vi "OpenMV.vi"(7 "JPG":refnum<vi>, 10 "queueName":string="PV_script", 11 "Console Reference":refnum<vi>) -> ()   [LabVIEW 2022 SP3]
panel:
  in  "Grab":bool
  in  "Snap":bool
  out "Image":picture
  out "Plots":T1
  in  "start":bool
  # "Camera View"
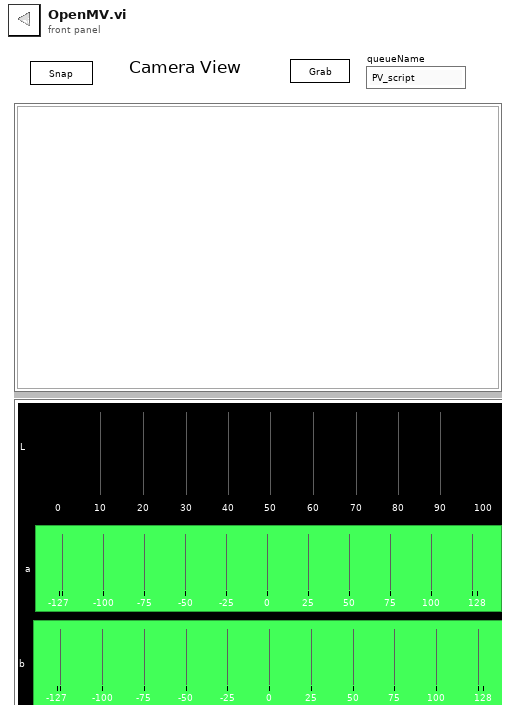
[diagram p1: front panel]
types:
  T1 = cluster{"L":dbl[], "a":cluster{i32, i32, dbl[]}, "b":cluster{i32, i32, dbl[]}}
  T2 = enum16{"read", "write pause", "write port", "write path", "write all"}
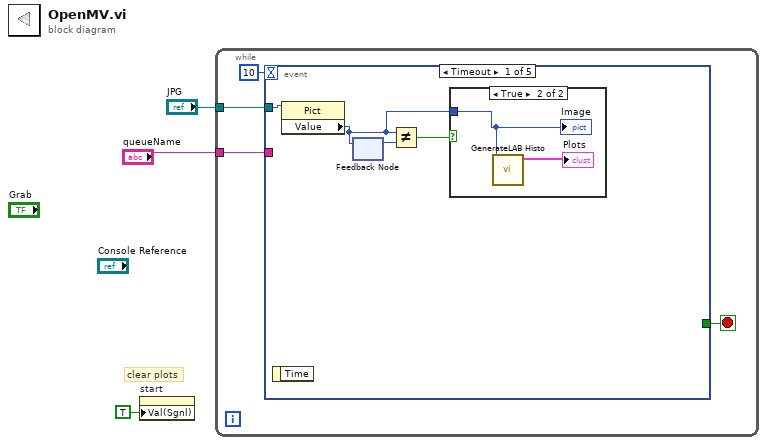
[diagram p0: block diagram]
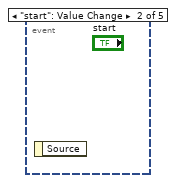
[diagram p3: hidden frame]
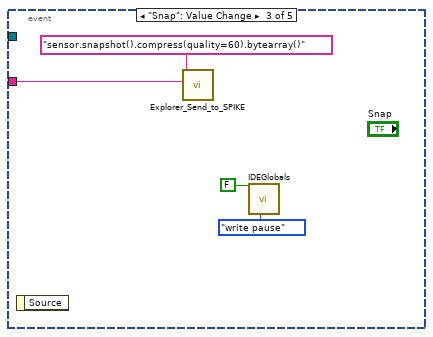
[diagram p4: hidden frame]
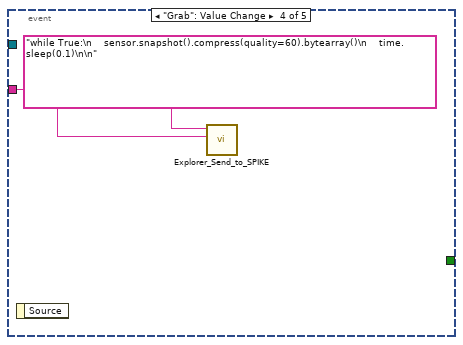
[diagram p5: hidden frame]
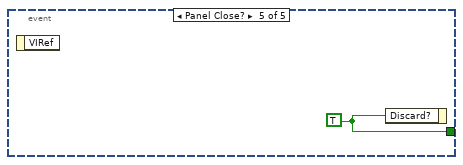
[diagram p6: hidden frame]
diagram:
  # "clear plots"
  n1 = property on="start" class="Bool (strict)"("Val(Sgnl)"=TRUE ("Value (Signaling)")) -> ()  [unwired: 2 in, 2 out]
  n2 = while {
    tunnel: "JPG" -> [w5]
    tunnel: "queueName" -> [w4]
    stop <- w6 stop-if-true
    n3 = event shown="[0] Timeout" {
      selector: _ -> [_ _ _ _ _]
      dyn-events: _ -> [_ _ _ _ _]
      timeout: 10 -> [_ _ _ _ _]
      tunnel: [_ _ _ _ w20] -> w6
      tunnel: w5 -> [w11 _ _ _ _]
      tunnel: w4 -> [_ _ w16 w18 _]
      event Timeout {
        n4 = event-data() -> ()  [unwired: 1 in, 1 out]
        n5 = property on="Property Node" class="Pict"(reference=w11) -> ("Value"=w8:picture)  [unwired: 1 in, 2 out]
        n6 = feedback #1() -> (w10:picture)  [unwired: 1 in]
        n7 = feedback-in #1(w8) -> ()
        n8 = Not Equal?(x=w8, y=w10) -> (x != y?=w9:bool)
        n9 = case shown="True" w9 {
          tunnel: w8 -> [_ w13]
          frame False {
          }
          frame True {
            n10 = call "GenerateLAB Histo.vi"("2D Picture"=w13) -> ("Plots"=→"Plots":T1)  [unwired: 9 in, 1 out]
            "Image" <- w13
          }
        }
      }
      event "start": Value Change {
        n11 = event-data() -> ()  [unwired: 1 in, 1 out]
      }
      event "Snap": Value Change {
        n12 = event-data() -> ()  [unwired: 1 in, 1 out]
        n13 = call "Explorer_Send_to_SPIKE.vi"("queueName"=w16, "python"="sensor.snapshot().compress(quality=60).bytearray()") -> ()  [unwired: 9 in, 1 out]
        n14 = call "IDEGlobals.vi"("task"=T2."write pause", "pause?"=FALSE) -> ()  [unwired: 7 in, 3 out]
      }
      event "Grab": Value Change {
        n15 = event-data() -> ()  [unwired: 1 in, 1 out]
        n16 = call "Explorer_Send_to_SPIKE.vi"("queueName"=w18, "python"="while True:\n    sensor.snapshot().compress(quality=60).bytearray()\n    time.sleep(0.1)\n\n") -> ()  [unwired: 9 in, 1 out]
      }
      event Panel Close? {
        w20 = TRUE ("Discard?")
        n17 = event-data() -> ()  [unwired: 1 in, 1 out]
        n18 = event-data("Discard?"=w20) -> ()  [unwired: 1 in, 1 out]
      }
    }
  }
